vi "DAQmx Create Channel (TEDS-AI-Temperature-Thermocouple).vi"(0 "task in":refnum<k21>, 1 "maximum value":dbl=100.0 format="%0.2f", 2 "minimum value":dbl format="%0.2f", 5 "physical channels":tag, 6 "cjc source":i32(ring)=10116 items=["Built-In"=10200, "Constant Value"=10116, "Channel"=10113], 7 "name to assign":string, 9 "units":i32(ring)=10143 items=["Deg C"=10143, "Deg F"=10144, "Kelvins"=10325, "Deg R"=10145, "From Custom Scale"=10065], 10 "cjc channel":refnum<k21>, 11 "error in":errorcluster, 14 "cjc value":dbl=25.0 format="%0.2f") -> (4 "task out":refnum<k21>, 15 "error out":errorcluster)   [LabVIEW 2013]
doc: "Creates channel(s) that use a thermocouple to measure temperature. You must configure the physical channel(s) with TEDS information to use this VI."
uses:
  C:/Program Files/National Instruments/LabVIEW 2013/resource/objmgr/daqmx.rc
panel:
  # "input limits"
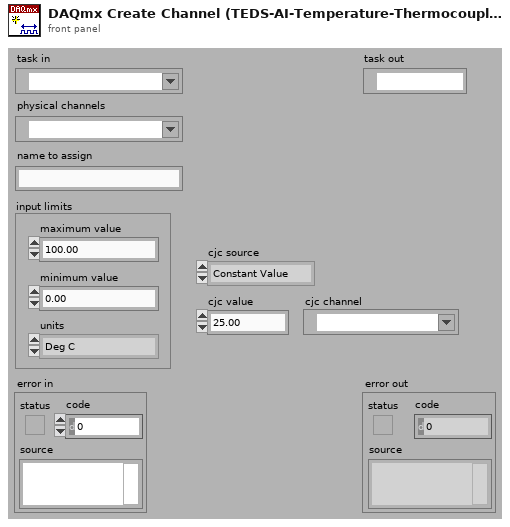
[diagram p1: front panel]
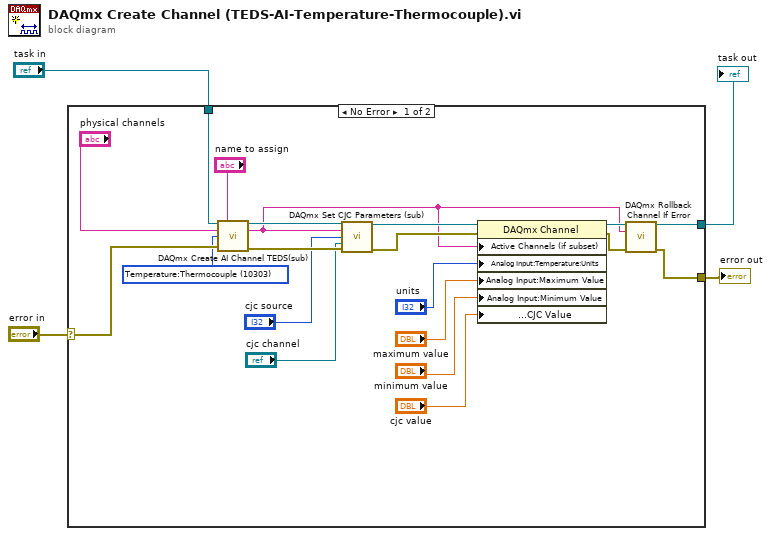
[diagram p0: block diagram]
diagram:
  n1 = case shown="No Error" "error in" {
    selector: "error in" -> [w23 w25]
    tunnel: [w7 w25] -> w4
    tunnel: "task in" -> [w24 w26]
    tunnel: [w8 w26] -> w1
    frame No Error {
      w5 = 10303 items=["Voltage"=10322, "Current"=10134, "More:Voltage:Custom with Excitation"=10323, "More:Current:Custom with Excitation"=10136, "Frequency"=10181, "Period"=10257, "Resistance"=10278, "Temperature:Thermocouple"=10303, "Temperature:Thermistor"=10302, "Temperature:RTD"=10301, "Temperature:Built-in Sensor"=10311, "Strain Gage"=10300, "LVDT"=10352, "RVDT"=10353, "Accelerometer:Voltage Input"=10355, "Accelerometer:Current Input"=10356, "Sound Pressure:Microphone"=10354, "TEDS"=12531] ("measurement type")
      n2 = call "DAQmx Create AI Channel TEDS(sub).vi"("task in"=w24, "virtual channel name"="name to assign", "physical channel name"="physical channels", "measurement type"=w5, "error in"=w23) -> ("task out"=w16:refnum<k21>, "channel names"=w6:string, "error out"=w15:errorcluster)  [unwired: 1 in, 7 out]
      n3 = call "DAQmx Set CJC Parameters (sub).vi"("task in"=w16, "thermocouple channel"=w6, "cjc source"="cjc source", "cjc channel"="cjc channel", "error in"=w15) -> ("task out"=w13:refnum<k21>, "error out"=w12:errorcluster)  [unwired: 9 out]
      n4 = property class="DAQmx Channel"(reference=w13, error in=w12, "Active Channels (if subset)"=w6, "Analog Input:Temperature:Units"="units", "Analog Input:Maximum Value"="maximum value", "Analog Input:Minimum Value"="minimum value", "Analog Input:Temperature:Thermocouple:CJC Value"="cjc value") -> (reference out=w10:refnum<k21>, error out=w9:errorcluster)
      n5 = call "DAQmx Rollback Channel If Error.vi"("task in"=w10, "channel names"=w6, "error in"=w9) -> ("task out"=w8:refnum<k21>, "error out"=w7:errorcluster)  [unwired: 11 out]
    }
    frame Error {
    }
  }
  "error out" <- w4
  "task out" <- w1
